vi "expCurveFit.vi"(11 "Array":i32[](array[numeric])) -> (1 "Decay Time":dbl, 3 "best fit":dynamicdata(graph))   [LabVIEW 2014]
doc: "This Program takes in an array of data, plots it, and computes the exponential fit. It also computes the decay time\n\nBryan Ghahremani - SID: 1135515\nKenneth Heide - SID: 1269429"
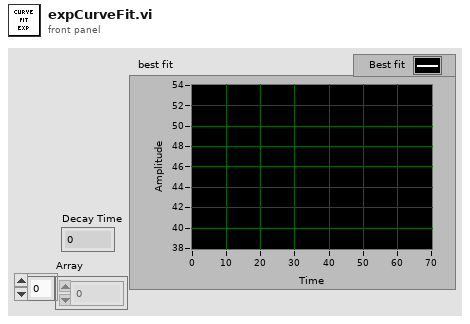
[diagram p1: front panel]
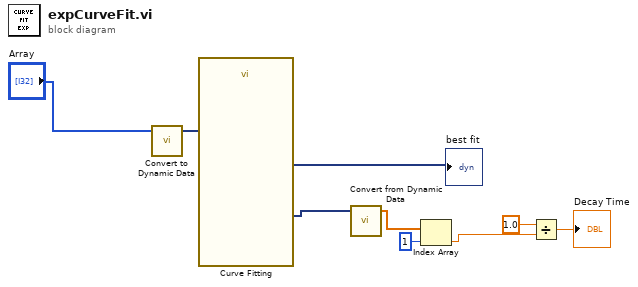
[diagram p0: block diagram]
diagram:
  n1 = call "Convert to Dynamic Data"("Array"="Array") -> ("Dynamic Data Type"=w9:dynamicdata)  [unwired: 3 in]
  n2 = call "Curve Fitting"("Signals"=w9) -> ("best fit"=→"best fit":dynamicdata, "non-linear coefficients"=w6:dynamicdata)  [unwired: 6 in, 3 out]
  n3 = call "Convert from Dynamic Data"("Dynamic Data Type"=w6) -> ("Array"=w5:dbl[])  [unwired: 3 in]
  n4 = Index Array(array=w5, index=1) -> (element=w3:dbl)
  n5 = Divide(x=1.0, y=w3) -> (x/y=→"Decay Time":dbl)
